vi "Free Space Path Loss.vi"(2 "Uplink Frequency (MHz)":dbl, 3 "Downlink Frequency (MHz)":dbl=20.0, 4 "distance (km)":dbl) -> (0 "Downlink Free Space Path Loss (dB)":dbl, 1 "Uplink Free Space Path Loss (dB)":dbl)   [LabVIEW 2015]
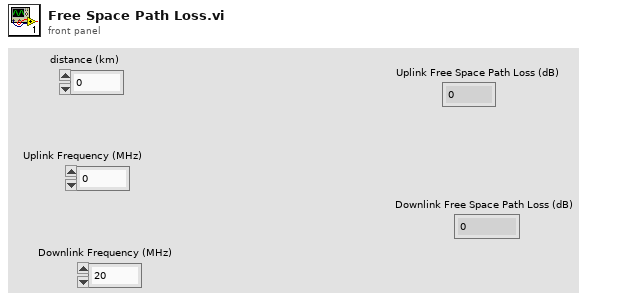
[diagram p1: front panel]
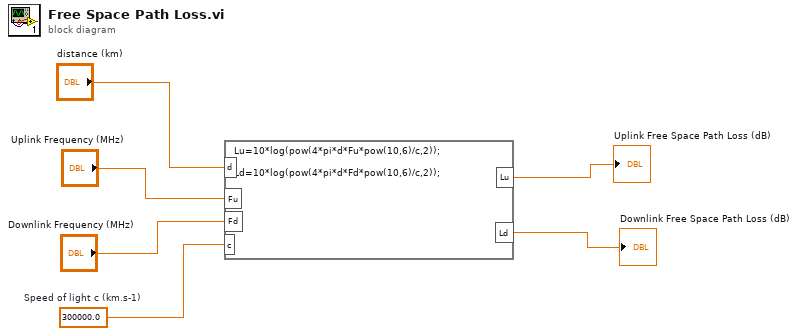
[diagram p0: block diagram]
diagram:
  w4 = 300000.0  # Speed of light c (km.s-1)
  n1 = formula code="Lu=10*log(pow(4*pi*d*Fu*pow(10,6)/c,2));\n\nLd=10*log(pow(4*pi*d*Fd*pow(10,6)/c,2));"("d"="distance (km)", "Fu"="Uplink Frequency (MHz)", "Fd"="Downlink Frequency (MHz)", "c"=w4) -> ("Lu"=→"Uplink Free Space Path Loss (dB)":dbl, "Ld"=→"Downlink Free Space Path Loss (dB)":dbl)
